vi "Configure Read File.vi"(0 "subVI":refnum<vi>, 2 "VI":refnum<vi>, 3 "ParentVI":refnum<vi>) -> (1 "Data Valid":bool)   [LabVIEW 2017]
doc: "Reads data from a LabVIEW measurement data file."
uses:
  <vilib>/express/express input/ExFileReadBlock.llb/ex_ReadFileGenericParams.ctl
  <vilib>/express/express shared/ExFile.llb/ex_FileGlobals.vi
panel:
  in  "always hostless warning":string="The present target will not have a host connected.  When run, this VI will return an error."
  in  "maybe hostless warning":string="The present target may not always have a host connected.  When running hostless, this VI will return an error."
  in  "delimiter string":string
  in  "Retrieve segments of original size":bool
  in  "absolute time":bool
  in  "relative time?":bool
  in  "Decimal point":enum32{". (dot)", ", (comma)"}(radio)
  in  "Delimiter":enum32{"tab", "comma"}(radio)
  in  "storage_format":enum32{"lvm", "tdm"}(radio)
  in  "File name":path=path "test.lvm"
  in  "File path":path
  in  "Unable to Load":string="Unable to Read from File"
  in  "Generic Params":T1
  in  "Read File Now":bool
  out "Sample data":string[][](table)
  in  "First column is time channel":bool
  in  "First row is channel names":bool
  in  "Start row of numeric data":i32=1 min=1
  in  "Read generic text files":bool
  in  "Help":bool
  in  "Ok":bool
  in  "Cancel":bool
  in  "Retrieve segments of specified size":bool
  in  "Samples":i32=1 min=1
  in  "Ask user to choose file":bool
  # "File Format"
  # "File Name"
  # "Action"
  # "Time Stamps"
  # "Segment Size"
  # "Generic Text File"
  # "Delimiter"
  # "Decimal Point"
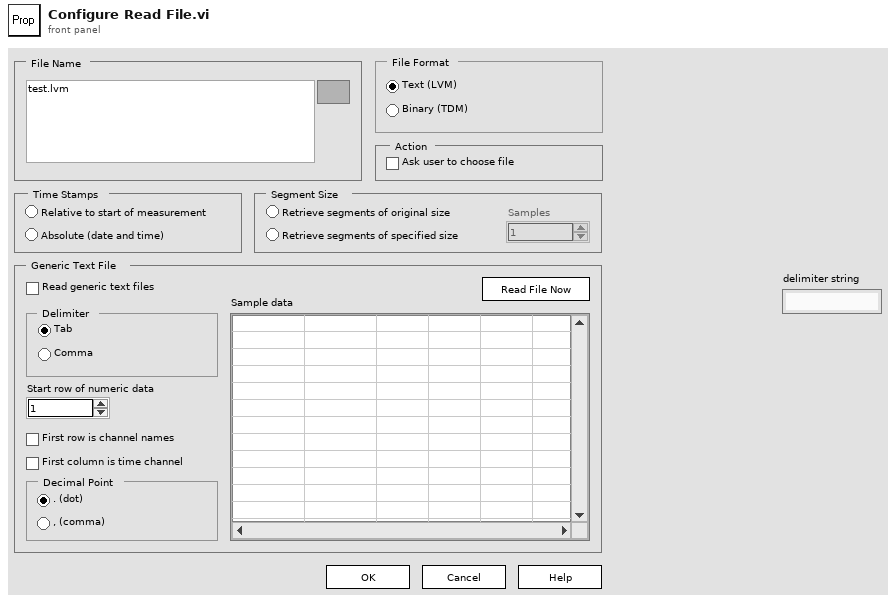
[diagram p1: front panel]
types:
  T1 = typedef "ex_ReadFileGenericParams.ctl" = cluster{"Delimiter":string, "First Row is Channel Names":bool, "First Column is Time Channel":bool, "Decimal Point":i32, "Start Row":i32}
  T2 = cluster{"Ctl Type":u16, "LV Block Ctl Label":string, "Wizard Ctl Label":string}[]
  T3 = typedef "propPageData.ctl" = cluster{"InstanceCtlRefs":refnum<vi>[], "ConfigDlgCtlRefs":refnum<vi>[], "Control Data":cluster{"Ctl Type":u16, "Instance Ctl Label":string, "Config Dialog Ctl Label":string}[], "viref Instance":refnum<vi>, "Types":i32[], "Config DialogVI":refnum<vi>}
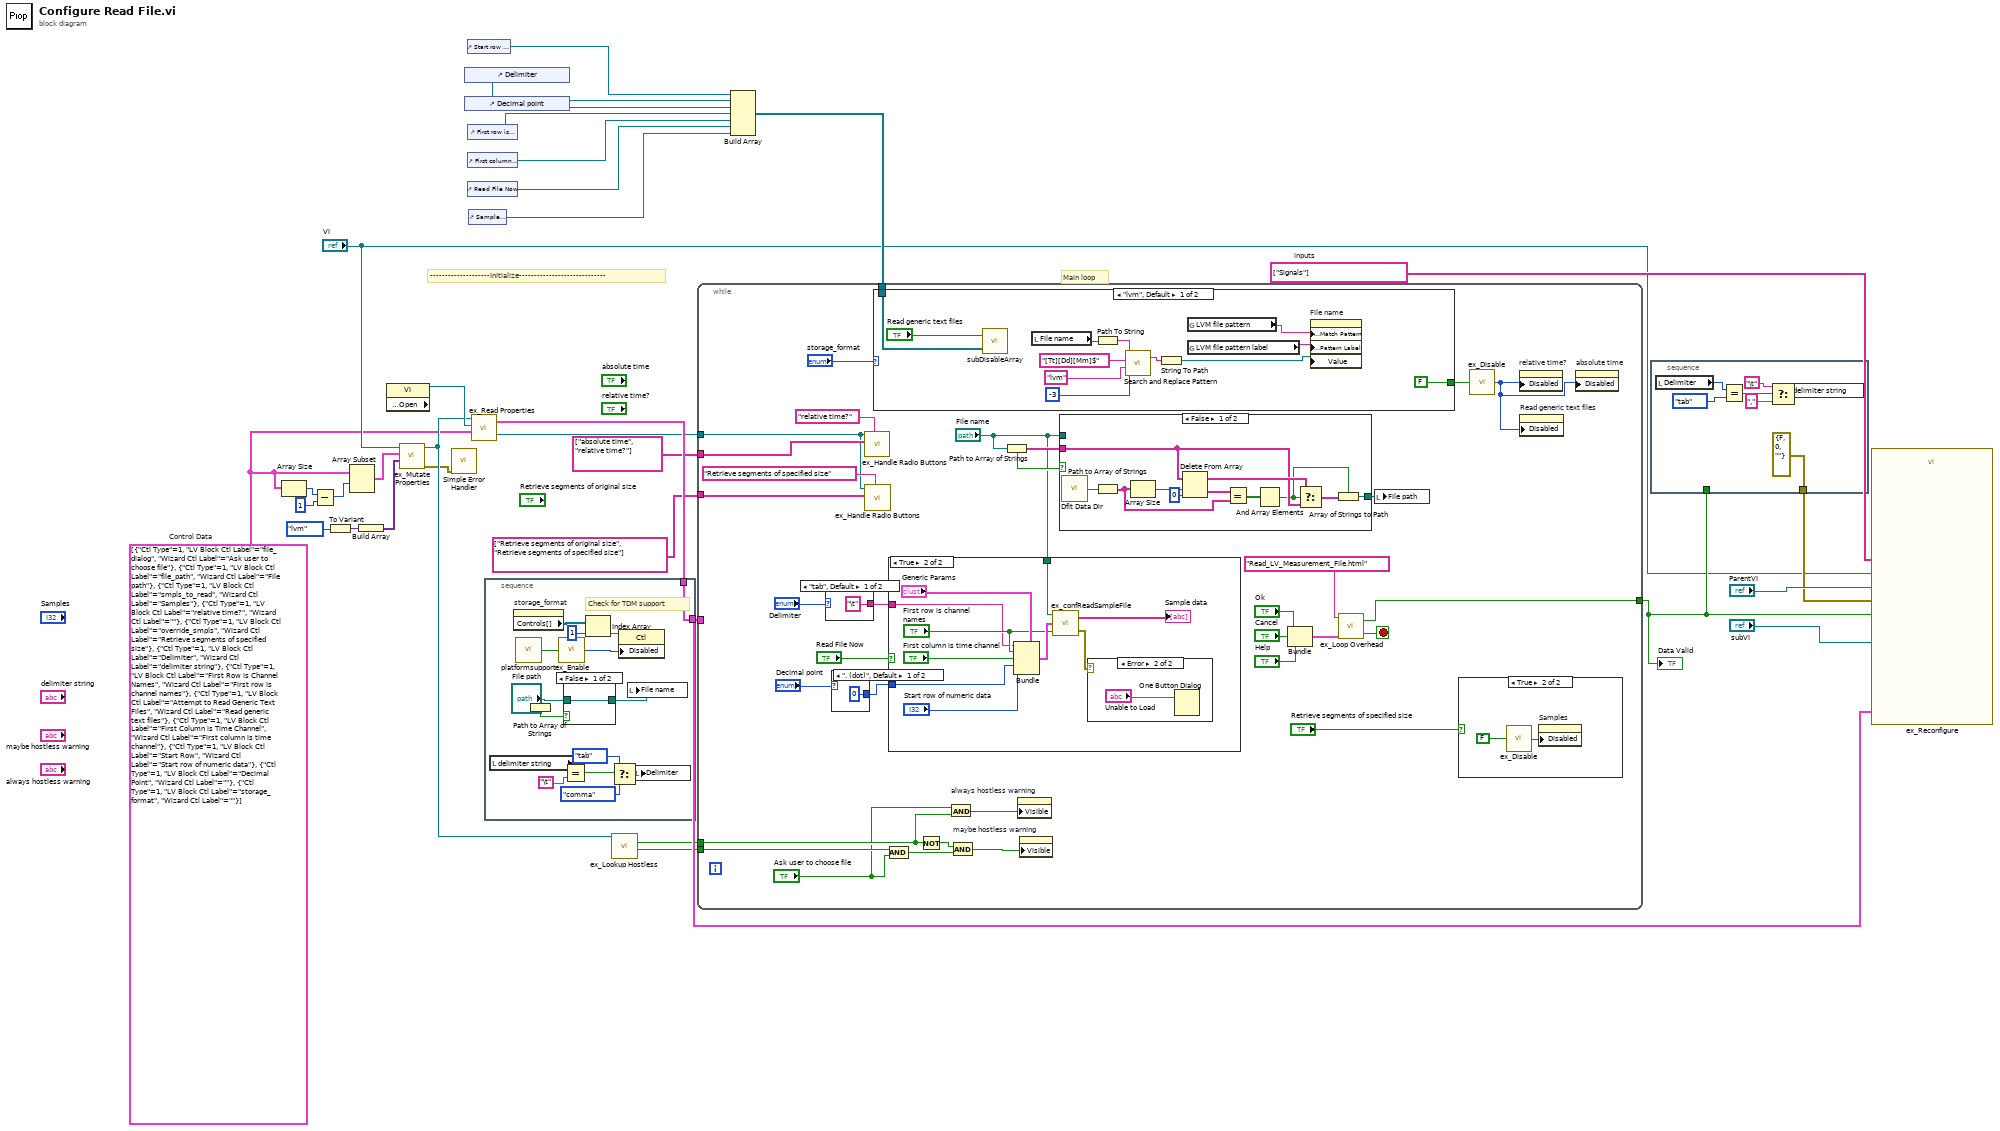
[diagram p0: block diagram]
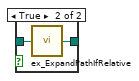
[diagram p2: hidden frame]
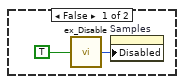
[diagram p3: hidden frame]
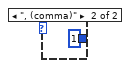
[diagram p4: hidden frame]
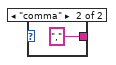
[diagram p5: hidden frame]
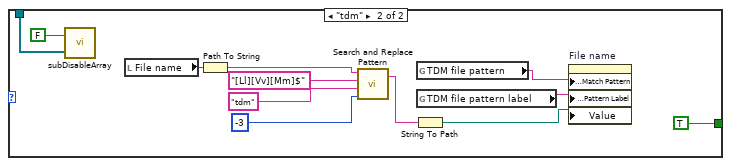
[diagram p6: hidden frame]
diagram:
  w16 = string[] ["Signals"]  # inputs
  w9 = T2 [{"Ctl Type"=1, "LV Block Ctl Label"="file_dialog", "Wizard Ctl Label"="Ask user to choose file"}, {"Ctl Type"=1, "LV Block Ctl Label"="file_path", "Wizard Ctl Label"="File path"}, {"Ctl Type"=1, "LV Block Ctl Label"="smpls_to_read", "Wizard Ctl Label"="Samples"}, {"Ctl Type"=1, "LV Block Ctl Label"="relative time?", "Wizard Ctl Label"=""}, {"Ctl Type"=1, "LV Block Ctl Label"="override_smpls", "Wizard Ctl Label"="Retrieve segments of specified size"}, {"Ctl Type"=1, "LV Block Ctl Label"="Delimiter", "Wizard Ctl Label"="delimiter string"}, {"Ctl Type"=1, "LV Block Ctl Label"="First Row is Channel Names", "Wizard Ctl Label"="First row is channel names"}, {"Ctl Type"=1, "LV Block Ctl Label"="Attempt to Read Generic Text Files", "Wizard Ctl Label"="Read generic text files"}, {"Ctl Type"=1, "LV Block Ctl Label"="First Column is Time Channel", "Wizard Ctl Label"="First column is time channel"}, {"Ctl Type"=1, "LV Block Ctl Label"="Start Row", "Wizard Ctl Label"="Start row of numeric data"}, {"Ctl Type"=1, "LV Block Ctl Label"="Decimal Point", "Wizard Ctl Label"=""}, {"Ctl Type"=1, "LV Block Ctl Label"="storage_format", "Wizard Ctl Label"=""}]  # Control Data
  # "--------------------Initialize-----------------------------"
  # "Main loop"
  n1 = Array Size(array=w9) -> (size(s)=w8:i32)
  n2 = Subtract(x=w8, y=1) -> (x-y=w6:i32)
  n3 = To Variant(anything=enum32{"lvm", "tdm"}."lvm" ("storage_format")) -> (Variant=w3:variant)
  n4 = Array Subset(array=w9, index=w6) -> (w5:T2)  [unwired: 1 in]
  n5 = Build Array(w3) -> (w2:variant[])
  n6 = property class="VI" props=["Front Panel Window:Open"]() -> (reference out=w32:refnum<vi>)  [unwired: 2 in, 2 out]
  n7 = call <vilib>:"ex_Mutate Properties.vi"("Control Values"=w2, "Control Data"=w5, "VI ref in"="VI") -> ("error out"=w1:errorcluster, "VI ref out"=w10:refnum<vi>)  [unwired: 7 out]
  n8 = call <vilib>:"Simple Error Handler.vi"("error in (no error)"=w1) -> ()  [unwired: 1 in, 8 out]
  n9 = control-ref of="Delimiter"() -> (w23:refnum<vi>)
  n10 = control-ref of="Decimal point"() -> (w24:refnum<vi>)
  n11 = control-ref of="Start row of numeric data"() -> (w22:refnum<vi>)
  n12 = control-ref of="First row is channel names"() -> (w28:refnum<vi>)
  n13 = control-ref of="First column is time channel"() -> (w27:refnum<vi>)
  n14 = control-ref of="Read File Now"() -> (w26:refnum<vi>)
  n15 = control-ref of="Sample data"() -> (w25:refnum<vi>)
  n16 = call <vilib>:"ex_Read Properties.vi"("Control Data"=w9, "viref Configuration Dialog"=w32, "viref Instance"=w10) -> ("viref Configuration Dialog out"=w21:refnum<vi>, "Output Cluster"=w29:T3)  [unwired: 1 in, 2 out]
  n17 = stacked-sequence {
    tunnel: w29 -> [w47]
    tunnel: [w47] -> w19
    frame #0 {
      # "Check for TDM support"
      n18 = local read "delimiter string"() -> (w33:string)
      n19 = property on="storage_format" class="RadioBtnsControl (strict)"() -> ("Controls[]"=w43:refnum<vi>[])  [unwired: 2 in, 2 out]
      n20 = call <vilib>:"platformsupport.vi"() -> ("TDM Support for Platform"=w39:bool)  [unwired: 1 out]
      n21 = Path to Array of Strings(0:"File path") -> (1:w45:bool)  [unwired: 1 out]
      n22 = call <vilib>:"ex_Enable.vi"("Enable?"=w39) -> ("Disabled Value"=w42:u8)
      n23 = Equal?(x=w33, y="\t") -> (x = y?=w37:bool)
      n24 = case shown="False" w45 {
        tunnel: "File path" -> [w48 w50]
        tunnel: [w48 w49] -> w46
        frame False {
        }
        frame True {
          n25 = call <vilib>:"ex_ExpandPathIfRelative.vi"("Path"=w50) -> ("Expanded path"=w49:path)  [unwired: 4 out]
        }
      }
      n26 = Index Array(array=w43, index=1) -> (element=w41:refnum<vi>)
      n27 = Select(t=enum32{"tab", "comma"}."tab" ("Delimiter"), s=w37, f=enum32{"tab", "comma"}."comma" ("Delimiter")) -> (s? t:f=w36:enum32{"tab", "comma"})
      n28 = property class="Ctl"(reference=w41, "Disabled"=w42) -> ()  [unwired: 1 in, 2 out]
      n29 = local write "File name"(w46) -> ()
      n30 = local write "Delimiter"(w36) -> ()
    }
  }
  n31 = call <vilib>:"ex_Lookup Hostless.vi"("VI RefNum for Context"=w10) -> ("Maybe Hostless"=w12:bool, "Always Hostless"=w13:bool)  [unwired: 1 in, 8 out]
  n32 = Build Array(w22, w23, w24, w28, w27, w26, w25) -> (w17:refnum<vi>[])
  n33 = while {
    tunnel: [w82] -> w15
    tunnel: w21 -> [w63]
    tunnel: string[] ["absolute time", "relative time?"] -> [w65]
    tunnel: w19 -> [_]
    tunnel: string[] ["Retrieve segments of original size", "Retrieve segments of specified size"] -> [w62]
    tunnel: w17 -> [w60]
    tunnel: w12 -> [w53]
    tunnel: w13 -> [w52]
    stop <- w81 stop-if-true
    n34 = case shown="\"tab\", Default" "Delimiter" {
      tunnel: ["\t" ","] -> w69
      frame "tab", Default {
      }
      frame "comma" {
      }
    }
    n35 = case shown="\". (dot)\", Default" "Decimal point" {
      tunnel: [0 1] -> w67
      frame ". (dot)", Default {
      }
      frame ", (comma)" {
      }
    }
    n36 = call <vilib>:"ex_Handle Radio Buttons.vi"("Boolean Control"="relative time?", "Radio Buttons"=w65, "VI refnum"=w63) -> ()  [unwired: 4 in, 5 out]
    n37 = call <vilib>:"ex_Handle Radio Buttons.vi"("Boolean Control"="Retrieve segments of specified size", "Radio Buttons"=w62, "VI refnum"=w63) -> ()  [unwired: 4 in, 5 out]
    n38 = case shown="\"lvm\", Default" "storage_format" {
      tunnel: w60 -> [w94 w106]
      tunnel: [FALSE ("Disable?") TRUE ("Disable?")] -> w59
      frame "lvm", Default {
        n39 = call <vilib>:"subDisableArray.vi"("Array"=w94, "Enable"="Read generic text files") -> ()
        n40 = local read "File name"() -> (w98:path)
        n41 = Path To String(path=w98) -> (string=w103:string)
        n42 = call <vilib>:"Search and Replace Pattern.vi"("string"=w103, "regular expression (\"\")"="[Tt][Dd][Mm]$" ("regular expression (\"\")"), "replace string (\"\")"="lvm" ("replace string (\"\")"), "offset (0)"=-3) -> ("result string"=w99:string)  [unwired: 2 out]
        n43 = String To Path(string=w99) -> (path=w95:path)
        n44 = global read "ex_FileGlobals.vi" "LVM file pattern"() -> (w97:string)
        n45 = global read "ex_FileGlobals.vi" "LVM file pattern label"() -> (w96:string)
        n46 = property on="File name" class="Path"("Browse Options:Match Pattern"=w97, "Browse Options:Pattern Label"=w96, "Value"=w95) -> ()  [unwired: 2 in, 2 out]
      }
      frame "tdm" {
        n47 = call <vilib>:"subDisableArray.vi"("Array"=w106, "Enable"=FALSE) -> ()
        n48 = local read "File name"() -> (w110:path)
        n49 = Path To String(path=w110) -> (string=w114:string)
        n50 = call <vilib>:"Search and Replace Pattern.vi"("string"=w114, "regular expression (\"\")"="[Ll][Vv][Mm]$" ("regular expression (\"\")"), "replace string (\"\")"="tdm" ("replace string (\"\")"), "offset (0)"=-3) -> ("result string"=w111:string)  [unwired: 2 out]
        n51 = String To Path(string=w111) -> (path=w107:path)
        n52 = global read "ex_FileGlobals.vi" "TDM file pattern"() -> (w109:string)
        n53 = global read "ex_FileGlobals.vi" "TDM file pattern label"() -> (w108:string)
        n54 = property on="File name" class="Path"("Browse Options:Match Pattern"=w109, "Browse Options:Pattern Label"=w108, "Value"=w107) -> ()  [unwired: 2 in, 2 out]
      }
    }
    n55 = And(x=w53, y="Ask user to choose file") -> (x .and. y?=w55:bool)
    n56 = case shown="True" "Read File Now" {
      tunnel: "File name" -> [_ w137]
      tunnel: w69 -> [_ w129]
      tunnel: w67 -> [_ w128]
      frame False {
      }
      frame True {
        n57 = Bundle(cluster="Generic Params", "Delimiter"=w129, "First Row is Channel Names"="First row is channel names", "First Column is Time Channel"="First column is time channel", "Decimal Point"=w128, "Start Row"="Start row of numeric data") -> (w135:T1)
        n58 = call <vilib>:"ex_confReadSampleFile.vi"("First Row is Channel Names"="First row is channel names", "Generic Params"=w135, "Expanded path"=w137) -> ("error out"=w130:errorcluster, "Sample Data"=→"Sample data":string[][])
        n59 = case shown="Error" w130 {
          frame No Error {
          }
          frame Error {
            n60 = One Button Dialog(message="Unable to Load") -> ()  [unwired: 2 out]
          }
        }
      }
    }
    n61 = Not(x=w52) -> (.not. x?=w54:bool)
    n62 = And(x="Ask user to choose file", y=w52) -> (x .and. y?=w56:bool)
    n63 = And(x=w54, y=w55) -> (x .and. y?=w57:bool)
    n64 = Path to Array of Strings(0:"File name") -> (1:w73:bool, 2:w74:string[])
    n65 = property on="always hostless warning" class="Str"("Visible"=w56) -> ()  [unwired: 2 in, 2 out]
    n66 = property on="maybe hostless warning" class="Str"("Visible"=w57) -> ()  [unwired: 2 in, 2 out]
    n67 = case shown="False" w73 {
      tunnel: [w118 w127] -> w75
      tunnel: "File name" -> [_ w127]
      tunnel: w74 -> [w117 _]
      frame False {
        n68 = call <vilib>:"Dflt Data Dir.vi"() -> ("App:Default Data Directory"=w119:path)
        n69 = Path to Array of Strings(0:w119) -> (2:w126:string[])  [unwired: 1 out]
        n70 = Array Size(array=w126) -> (size(s)=w120:i32)
        n71 = Delete From Array(array=w117, length=w120, index=0) -> (deleted portion=w125:string[], array with subset deleted=w124:string[])
        n72 = Equal?(x=w125, y=w126) -> (x = y?=w122:bool[])
        n73 = And Array Elements(Boolean array=w122) -> (logical AND=w116:bool)
        n74 = Select(t=w124, s=w116, f=w117) -> (s? t:f=w123:string[])
        n75 = Array of Strings to Path(0:w123, 1:w116) -> (2:w118:path)
      }
      frame True {
      }
    }
    n76 = Bundle("Ok"="Ok", "Cancel"="Cancel", "Help"="Help") -> (w77:cluster{"Ok":bool, "Cancel":bool, "Help":bool})  [unwired: 1 out]
    n77 = call <vilib>:"ex_Loop Overhead.vi"("Bottom Button Bar"=w77, "Help string to search for"="Read_LV_Measurement_File.html") -> ("Loop Terminator"=w81:bool, "Data Valid"=w82:bool)  [unwired: 1 in, 1 out]
    n78 = local write "File path"(w75) -> ()
    n79 = case shown="True" "Retrieve segments of specified size" {
      frame False {
        n80 = call <vilib>:"ex_Disable.vi"("Disable?"=TRUE) -> ("Disabled value"=w85:u8)
        n81 = property on="Samples" class="DigNum (strict)"("Disabled"=w85) -> ()  [unwired: 2 in, 2 out]
      }
      frame True {
        n82 = call <vilib>:"ex_Disable.vi"("Disable?"=FALSE) -> ("Disabled value"=w87:u8)
        n83 = property on="Samples" class="DigNum (strict)"("Disabled"=w87) -> ()  [unwired: 2 in, 2 out]
      }
    }
    n84 = call <vilib>:"ex_Disable.vi"("Disable?"=w59) -> ("Disabled value"=w58:u8)
    n85 = property on="relative time?" class="Bool (strict)"("Disabled"=w58) -> ()  [unwired: 2 in, 2 out]
    n86 = property on="Read generic text files" class="Bool (strict)"("Disabled"=w58) -> ()  [unwired: 2 in, 2 out]
    n87 = property on="absolute time" class="Bool (strict)"("Disabled"=w58) -> ()  [unwired: 2 in, 2 out]
  }
  "Data Valid" <- w15
  n88 = stacked-sequence {
    tunnel: w15 -> [_]
    tunnel: [errorcluster {"status"=FALSE, "code"=0, "source"=""} ("error out")] -> w14
    frame #0 {
      n89 = local read "Delimiter"() -> (w143:enum32{"tab", "comma"})
      n90 = Equal?(x=w143, y=enum32{"tab", "comma"}."tab" ("Delimiter")) -> (x = y?=w145:bool)
      n91 = Select(t="\t", s=w145, f=",") -> (s? t:f=w141:string)
      n92 = local write "delimiter string"(w141) -> ()
    }
  }
  n93 = call <vilib>:"ex_Reconfigure.vi"("VI refnum"="VI", "Parent VI refnum"="ParentVI", "Data Valid"=w15, "subVI refnum"="subVI", "error in"=w14, "Inputs/Outputs to Grow"=w16, "Props Cluster"=w19) -> ()  [unwired: 6 in, 15 out]
